vi "Task Awaiter.vi"(8 "error in (no error)":errorcluster, 10 "Timeout":i32=-1, 11 "Task":refnum<k24>) -> (0 "error out":errorcluster, 2 "Timeout":bool, 3 "Task":refnum<k24>)   [LabVIEW 2020, in "WebView2 Control.xctl"]
uses:
  WebView2 Control.xctl
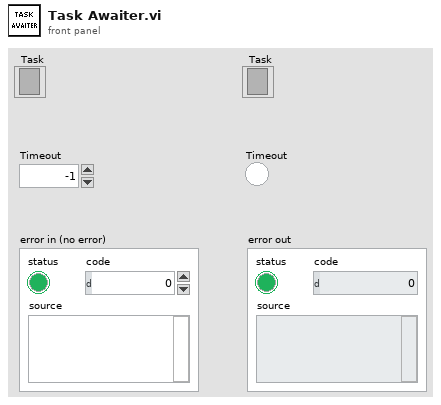
[diagram p1: front panel]
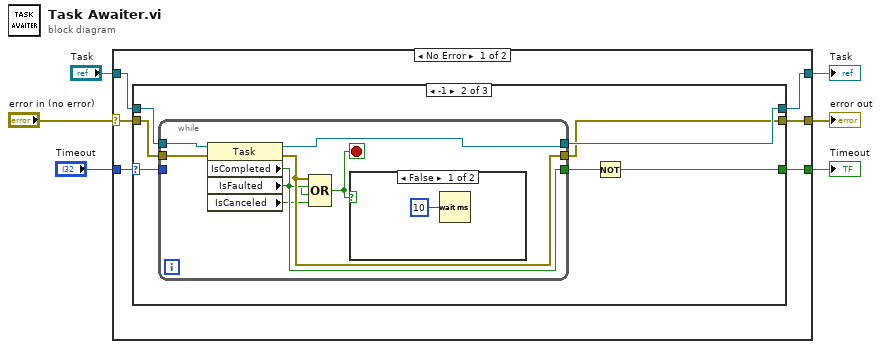
[diagram p0: block diagram]
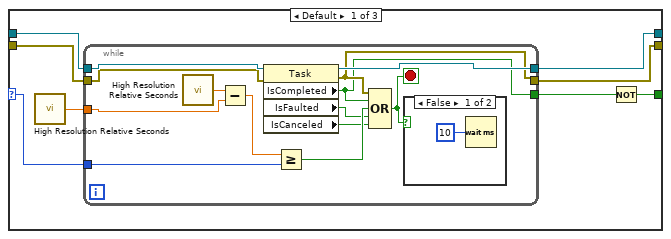
[diagram p2: hidden frame]
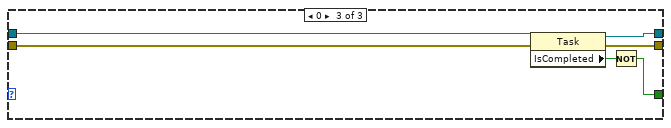
[diagram p5: hidden frame]
diagram:
  n1 = case shown="No Error" "error in (no error)" {
    selector: "error in (no error)" -> [w11 w58]
    tunnel: "Task" -> [w12 w57]
    tunnel: "Timeout" -> [w10 _]
    tunnel: [w9 w58] -> w3
    tunnel: [w8 w57] -> w2
    tunnel: [w7 _] -> w1
    frame No Error {
      n2 = case shown="-1" w10 {
        selector: w10 -> [w17 w38 _]
        tunnel: w12 -> [w20 w41 w56]
        tunnel: w11 -> [w19 w40 w55]
        tunnel: [w18 w39 w54] -> w8
        tunnel: [w16 w37 w51] -> w9
        tunnel: [w13 w35 w52] -> w7
        frame Default {
          n3 = call <vilib>:"High Resolution Relative Seconds.vi"() -> ("relative seconds"=w15:dbl)
          n4 = while {
            tunnel: w20 -> [w33]
            tunnel: w19 -> [w32]
            tunnel: [w31] -> w18
            tunnel: w15 -> [w29]
            tunnel: w17 -> [w27]
            tunnel: [w25] -> w16
            tunnel: [w24] -> w14
            stop <- w21 stop-if-true
            n5 = call <vilib>:"High Resolution Relative Seconds.vi"() -> ("relative seconds"=w30:dbl)
            n6 = Subtract(x=w30, y=w29) -> (x-y=w28:dbl)
            n7 = property class="Task"(reference=w33, error in=w32) -> (reference out=w31:refnum<k24>, error out=w25:errorcluster, "IsCompleted"=w24:bool, "IsFaulted"=w23:bool, "IsCanceled"=w22:bool)
            n8 = Greater Or Equal?(x=w28, y=w27) -> (x >= y?=w26:bool)
            n9 = Compound Arithmetic op=OR(w25, w24, w26, w23, w22) -> (w21:bool)
            n10 = case shown="False" w21 {
              frame False {
                n11 = Wait (ms)(milliseconds to wait=u32 10) -> ()  [unwired: 1 out]
              }
              frame True {
              }
            }
          }
          n12 = Not(x=w14) -> (.not. x?=w13:bool)
        }
        frame -1 {
          n13 = while {
            tunnel: w41 -> [w49]
            tunnel: w40 -> [w48]
            tunnel: [w47] -> w39
            tunnel: w38 -> [_]
            tunnel: [w46] -> w37
            tunnel: [w45] -> w36
            stop <- w42 stop-if-true
            n14 = property class="Task"(reference=w49, error in=w48) -> (reference out=w47:refnum<k24>, error out=w46:errorcluster, "IsCompleted"=w45:bool, "IsFaulted"=w44:bool, "IsCanceled"=w43:bool)
            n15 = Compound Arithmetic op=OR(w46, w45, w44, w43) -> (w42:bool)
            n16 = case shown="False" w42 {
              frame False {
                n17 = Wait (ms)(milliseconds to wait=u32 10) -> ()  [unwired: 1 out]
              }
              frame True {
              }
            }
          }
          n18 = Not(x=w36) -> (.not. x?=w35:bool)
        }
        frame 0 {
          n19 = property class="Task"(reference=w56, error in=w55) -> (reference out=w54:refnum<k24>, error out=w51:errorcluster, "IsCompleted"=w53:bool)
          n20 = Not(x=w53) -> (.not. x?=w52:bool)
        }
      }
    }
    frame Error {
    }
  }
  "error out" <- w3
  "Task" <- w2
  "Timeout" <- w1
